vi "Switch Handle Test Complete.vi"(6 "Quick Mode (F)":bool, 8 "error in (no error)":errorcluster, 9 "Test Parameters":T1, 11 "Queue":refnum<queue>) -> (0 "error out":errorcluster)   [LabVIEW 2011]
uses:
  TypeDefs/Switch Queue Cluster.ctl
  TypeDefs/Switch Test Parameters.ctl
  TypeDefs/Switch Stimulus Parameters.ctl
  TypeDefs/Switch Type.ctl
  TypeDefs/Switch Instrument Info.ctl
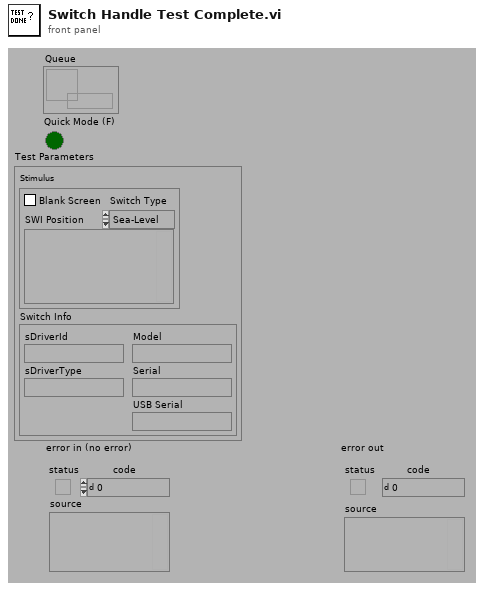
[diagram p1: front panel]
types:
  T1 = typedef "Switch Test Parameters.ctl" = cluster{"Stimulus":T2, "Switch Info":T4}
  T2 = typedef "Switch Stimulus Parameters.ctl" = cluster{"Blank Screen":bool, "SWI Position":variant, "Switch Type":T3}
  T3 = typedef "Switch Type.ctl" = enum16{"Sea-Level", "Simulator", "SI-0206-SW", "SI-0309-SW", "SI-0310-SW", "Front End"}
  T4 = typedef "Switch Instrument Info.ctl" = cluster{"sDriverId":string, "sDriverType":string, "Model":string, "Serial":string, "USB Serial":string}
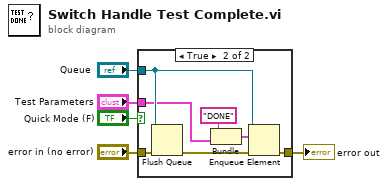
[diagram p0: block diagram]
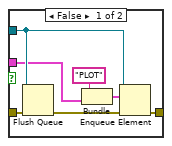
[diagram p2: hidden frame]
diagram:
  n1 = case shown="True" "Quick Mode (F)" {
    tunnel: [w12 w19] -> w5
    tunnel: "Queue" -> [w8 w15]
    tunnel: "error in (no error)" -> [w9 w16]
    tunnel: "Test Parameters" -> [w6 w13]
    frame False {
      n2 = Flush Queue(queue=w8, error in (no error)=w9) -> (error out=w7:errorcluster)  [unwired: 2 out]
      n3 = Bundle("PLOT", "Test Parameters"=w6) -> (w10:cluster{string, "Test Parameters":T1})  [unwired: 1 out]
      n4 = Enqueue Element(queue=w8, element=w10, error in (no error)=w7) -> (error out=w12:errorcluster)  [unwired: 3 out]
    }
    frame True {
      n5 = Flush Queue(queue=w15, error in (no error)=w16) -> (error out=w14:errorcluster)  [unwired: 2 out]
      n6 = Bundle("DONE", "Test Parameters"=w13) -> (w17:cluster{string, "Test Parameters":T1})  [unwired: 1 out]
      n7 = Enqueue Element(queue=w15, element=w17, error in (no error)=w14) -> (error out=w19:errorcluster)  [unwired: 3 out]
    }
  }
  "error out" <- w5
